vi "Stop Core.vi"(10 "final error code":i32, 11 "Network Actor in":refnum<class "Network Actor.lvclass">) -> (3 "Network Actor out":refnum<class "Network Actor.lvclass">)   [LabVIEW 2014, in "Network Actor Library.lvlib" / "Network Actor.lvclass"]
doc: "(<B>Filename</B>: Actor Framework.lvlib:Actor.lvclass:Stop Core.vi)\n\nDefines what the actor does before it stops. Use the <B>final error code</B> input to determine whether the actor shut down in response to an error.\n\nBy default, this method does nothing. A descendant class may override it to define behavior, such as shutting down any processes the actor initiated in its override of the Actor Core method."
uses:
  Network Actor.lvclass
  SuperActor/SuperActor.lvclass/SuperActor.ctl
  Network Actor.lvclass/Network Actor.ctl
  SuperActor/Read Log Session.vi
  SuperActor/SuperActor.lvclass
  <userlib>/_Session Fwk/Session - Root.lvclass
  reusable/Session APIs/Session Log/System Log.lvclass
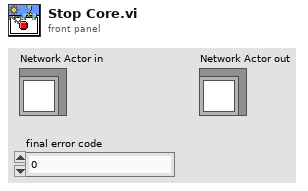
[diagram p1: front panel]
types:
  T1 = typedef "Session - Root.lvclass/Session Handle.ctl" = refnum<data-value>
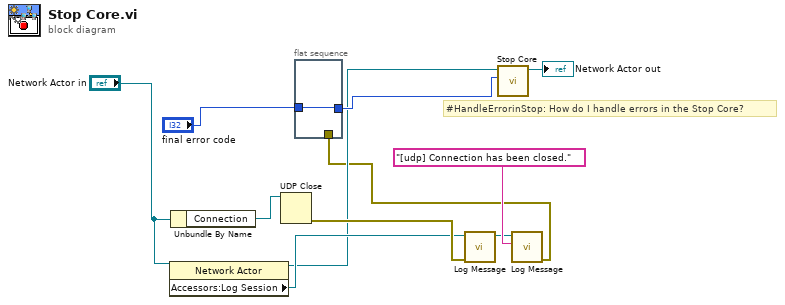
[diagram p0: block diagram]
diagram:
  # "#HandleErrorinStop: How do I handle errors in the Stop Core?"
  n1 = property class="Network Actor"(reference="Network Actor in") -> (reference out=w2:refnum<class "Network Actor.lvclass">, "Accessors:Log Session"=w6:T1)  [unwired: 1 in, 1 out]
  n2 = Unbundle By Name("Network Actor in") -> ("Connection"=w11:refnum<k16>)
  n3 = UDP Close(connection ID=w11) -> (error out=w9:errorcluster)  [unwired: 1 in, 1 out]
  n4 = flat-sequence {
    tunnel: "final error code" -> [w12]
    tunnel: [w12] -> w3
    tunnel: w1 -> [_]
    frame #0 {
    }
  }
  n5 = call "Log Message.vi"("error in"=w9, "session in"=w6) -> ("session out"=w8:T1)  [unwired: 8 in, 1 out]
  n6 = call-parent "Stop Core.vi"("final error code"=w3, "Ex Nested in"=w2) -> ("Ex Nested out"=→"Network Actor out":refnum<class "Network Actor.lvclass">)  [unwired: 9 in]
  n7 = call "Log Message.vi"("MSG In"="[udp] Connection has been closed.", "session in"=w8) -> ("error out"=w1:errorcluster)  [unwired: 8 in, 1 out]
